vi "Actor Core.vi"(8 "error in":errorcluster, 11 "DMM Driver in":refnum<class "DMM Driver.lvclass">) -> (0 "error out":errorcluster, 3 "Actor out":refnum<class "Actor.lvclass">)   [LabVIEW 2020, in "DMM Driver.lvclass"]
doc: "(<B>Filename</B>: Actor Framework.lvlib:Actor.lvclass:Actor Core.vi)\n\nReceives messages to the actor, reacts to them, and initiates any error handling that may shut the actor down.\n\nDescendant classes may override this VI to append parallel tasks for the actor to complete while it handles messages. Overrides use the Call Parent Method node."
uses:
  DMM Driver.lvclass
  C:/Program Files (x86)/National Instruments/LabVIEW 2020/vi.lib/ActorFramework/Actor/Actor.lvclass
  <vilib>/ActorFramework/Actor/Actor.lvclass
  DMM Driver.lvclass/DMM Driver.ctl
  <vilib>/ActorFramework/Actor/Actor.lvclass/Actor.ctl
  <vilib>/ActorFramework/Message Enqueuer/Message Enqueuer.lvclass/Message Enqueuer.ctl
  <vilib>/ActorFramework/Message Enqueuer/Init from Existing Queue.vi
  <vilib>/ActorFramework/Message Enqueuer/Enqueue.vi
  <vilib>/ActorFramework/Stop Msg/Stop Msg.lvclass
  C:/Program Files (x86)/National Instruments/LabVIEW 2020/vi.lib/ActorFramework/Message/Message.lvclass
  DMM Driver Messages/Init DMM Msg/Init DMM Msg.lvclass
  DMM Driver Messages/Read DMM Msg/Read DMM Msg.lvclass
  DMM Driver Messages/Close DMM Msg/Close DMM Msg.lvclass
  DMM Driver Messages/Reset DMM Msg/Reset DMM Msg.lvclass
  <vilib>/ActorFramework/Message Priority Queue/Priority Enqueue.vi
  <vilib>/ActorFramework/Message Enqueuer/Message Enqueuer.lvclass
panel:
  out "Data":dbl
  in  "Reset DMM":bool
  in  "Stop Loop":bool
  in  "Close DMM":bool
  in  "Read DMM":bool
  in  "Init DMM":bool
  in  "Stop Button":bool
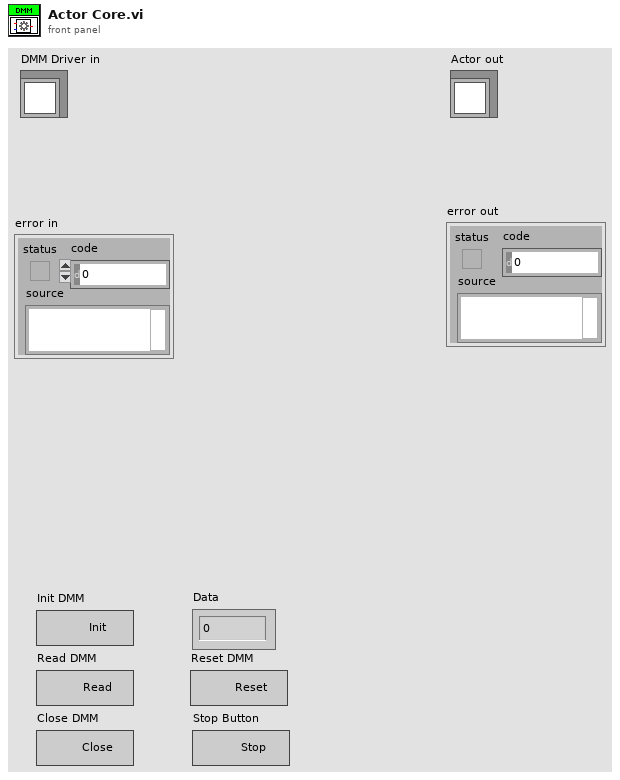
[diagram p1: front panel]
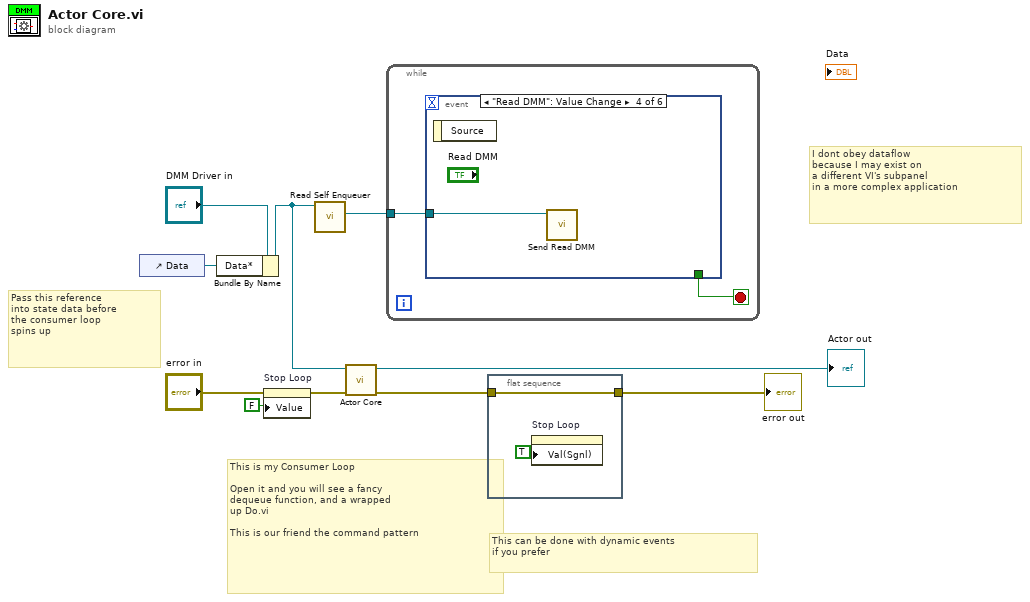
[diagram p0: block diagram]
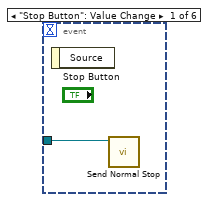
[diagram p2: hidden frame]
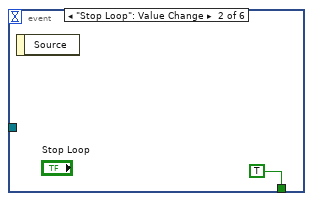
[diagram p3: hidden frame]
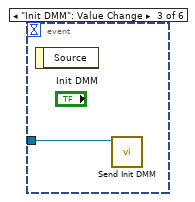
[diagram p4: hidden frame]
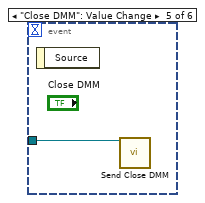
[diagram p5: hidden frame]
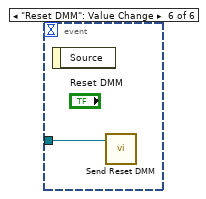
[diagram p6: hidden frame]
diagram:
  # "This is my Consumer Loop\n\nOpen it and you will see a fancy\ndequeue function, and a wrapped\nup Do.vi\n\nThis is our friend the command pattern"
  # "This can be done with dynamic events\nif you prefer"
  # "Pass this reference\ninto state data before\nthe consumer loop\nspins up"
  # "I dont obey dataflow\nbecause I may exist on\na different VI's subpanel\nin a more complex application"
  n1 = control-ref of="Data"() -> (w1:refnum<vi>)
  n2 = Bundle By Name(cluster="DMM Driver in", "Data*"=w1) -> (w2:refnum<class "DMM Driver.lvclass">)
  n3 = property on="Stop Loop" class="Bool (strict)"(error in="error in", "Value"=FALSE ("Stop Loop")) -> (error out=w7:errorcluster)  [unwired: 1 in, 1 out]
  n4 = call <vilib>:"Read Self Enqueuer.vi"("Actor"=w2) -> ("Self Enqueuer"=w9:refnum<class "Message Enqueuer.lvclass">)  [unwired: 10 in]
  n5 = call-parent "Actor Core.vi"("error in"=w7, "Actor in"=w2) -> ("error out"=w5:errorcluster, "Actor out"=→"Actor out":refnum<class "Actor.lvclass">)  [unwired: 8 in]
  n6 = while {
    tunnel: w9 -> [w12]
    stop <- w11 stop-if-true
    n7 = event shown="[3] \"Read DMM\": Value Change" {
      selector: _ -> [_ _ _ _ _ _]
      dyn-events: _ -> [_ _ _ _ _ _]
      timeout: _ -> [_ _ _ _ _ _]
      tunnel: w12 -> [w13 _ w15 w16 w17 w18]
      tunnel: [_ TRUE _ _ _ _] -> w11
      event "Stop Button": Value Change {
        n8 = event-data() -> ()  [unwired: 1 in, 1 out]
        n9 = call <vilib>:"Send Normal Stop.vi"("Message Enqueuer"=w13) -> ()  [unwired: 10 in, 1 out]
      }
      event "Stop Loop": Value Change {
        n10 = event-data() -> ()  [unwired: 1 in, 1 out]
      }
      event "Init DMM": Value Change {
        n11 = event-data() -> ()  [unwired: 1 in, 1 out]
        n12 = call "Send Init DMM.vi"("Message Enqueuer"=w15) -> ()  [unwired: 9 in, 2 out]
      }
      event "Read DMM": Value Change {
        n13 = event-data() -> ()  [unwired: 1 in, 1 out]
        n14 = call "Send Read DMM.vi"("Message Enqueuer"=w16) -> ()  [unwired: 9 in, 2 out]
      }
      event "Close DMM": Value Change {
        n15 = event-data() -> ()  [unwired: 1 in, 1 out]
        n16 = call "Send Close DMM.vi"("Message Enqueuer"=w17) -> ()  [unwired: 9 in, 2 out]
      }
      event "Reset DMM": Value Change {
        n17 = event-data() -> ()  [unwired: 1 in, 1 out]
        n18 = call "Send Reset DMM.vi"("Message Enqueuer"=w18) -> ()  [unwired: 9 in, 2 out]
      }
    }
  }
  n19 = flat-sequence {
    tunnel: [w20] -> w4
    tunnel: w5 -> [w20]
    frame #0 {
      n20 = property on="Stop Loop" class="Bool (strict)"("Val(Sgnl)"=TRUE ("Value (Signaling)")) -> ()  [unwired: 2 in, 2 out]
    }
  }
  "error out" <- w4
